vi "Drive Controller.vi"(8 "error in":errorcluster) -> ()   [LabVIEW 2020]
doc: "This VI executes continuously carrying out the current operation and responding to updates or new operation requests. It will often contain the timing or control code that is difficult to place directly in TeleOp. This VI generally opens all sensors and motors and isolates the rest of the robot code from knowing implementation details of how the operations are carried out."
uses:
  Drive Operations.ctl
  Drive Setpoints.ctl
  <vilib>/Rock Robotics/WPI/SafetyOutput/WPI_SafetyOutputConfigMenu.ctl
  <vilib>/Rock Robotics/WPI/RobotDrive/WPI_RobotDriveOpen2MotorWithExistingMotors.vi
  <vilib>/Rock Robotics/WPI/Framework/Completion Status.ctl
panel:
  in  "Interactive Values":T1
  in  "Buttons":cluster{"Execute Cmd":bool, "Abort Cmd":bool}
  out "Command Timing":cluster{"Start Time (ms)":u32, "Iterations":i32}
  out "Status":T3
  out "Setpoints":T4(graph)
  out "Current\nCmd":string
  # "Tip: The graph shows the motor setpoints. It may also be helpful to observe inputs and sensor values.\nYou may also want to display tuning or debugging controls."
  # "Interactive Command: You may fill in the settings for a command\nand schedule it with the Execute button. You can observe and abort\nany command while fine tuning the code for the controller."
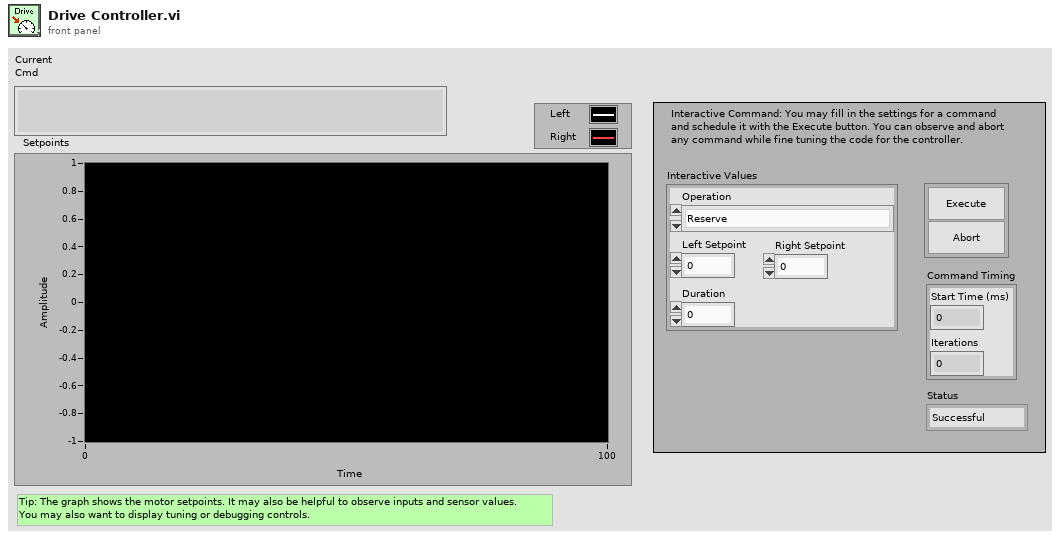
[diagram p1: front panel]
types:
  T1 = typedef "Drive Setpoints.ctl" = cluster{"Operation":T2, "Left Setpoint":dbl, "Right Setpoint":dbl, "Duration":dbl}
  T2 = typedef "Drive Operations.ctl" = enum16{"Reserve", "Read Current", "Immediate", "Drive for Time", "Drive for Distance"}
  T3 = typedef "Completion Status.ctl" = enum16{"Successful", "Aborted", "Incomplete"}
  T4 = cluster{"Left Setpoint":dbl, "Right Setpoint":dbl}
  T5 = typedef "WPI_SafetyOutputConfigMenu.ctl" = enum16{"Enable", "Disable"}
  T6 = typedef "WPI_MotorControlDeviceRef.ctl" = cluster{"DeviceStatus":errorcluster, "Type":T7, "PWM":cluster{"PWM Channel":T8, "DeadBand":T9}, "CAN":cluster{"Device Number":u8, "SetOutput VI Ref":variant, "GetOutput VI Ref":variant, "Enable VI Ref":variant, "Disable VI Ref":variant, "Data":variant}, "Invert":bool, "DIO PWM":cluster{"PWM \"Enable\" Channel":T8, "DIOChannel":T10, "PWM Rate":dbl}}
  T7 = typedef "WPI_MotorControlType.ctl" = enum16{"PWM", "CAN", "DIO PWM"}
  T8 = typedef "FPGA_DIOPWMChannel.ctl" = enum8{"PWM 0", "PWM 1", "PWM 2", "PWM 3", "PWM 4", "PWM 5", "PWM 6", "PWM 7", "PWM 8", "PWM 9", "PWM MXP 0", "PWM MXP 1", "PWM MXP 2", "PWM MXP 3", "PWM MXP 4", "PWM MXP 5", "PWM MXP 6", "PWM MXP 7", "PWM MXP 8", "PWM MXP 9", "Invalid"}
  T9 = typedef "WPI_PWMDeadband.ctl" = cluster{"Name":string, "maxPositivePwm":i32, "minPositivePwm":i32, "centerPwm":i32, "maxNegativePwm":i32, "minNegativePwm":i32, "angularRange":u16}
  T10 = typedef "FPGA_DIOChannel.ctl" = enum8{"DIO 0", "DIO 1", "DIO 2", "DIO 3", "DIO 4", "DIO 5", "DIO 6", "DIO 7", "DIO 8", "DIO 9", "DIO MXP 0", "DIO MXP 1", "DIO MXP 2", "DIO MXP 3", "DIO MXP 4", "DIO MXP 5", "DIO MXP 6", "DIO MXP 7", "DIO MXP 8", "DIO MXP 9", "DIO MXP 10", "DIO MXP 11", "DIO MXP 12", "DIO MXP 13", "DIO MXP 14", "DIO MXP 15", "SPI Port CS1", "SPI Port CS2", "SPI Port CS3", "SPI Port MISO", "SPI Port MOSI", "Invalid"}
  T11 = typedef "WPI_RobotDriveDevRef.ctl" = cluster{"DevStatus":errorcluster, "Motors[]":T6[], "Square Inputs":bool, "Max Output":dbl}
  T12 = typedef "Command Status Info.ctl" = cluster{"Name":string, "Status":T3, "notifier out":T13}
  T13 = typedef "Completion Notifier.ctl" = refnum<notifier>
  T14 = cluster{"SubSystem Data":T1, cluster{"Start Time (ms)":u32, "Iterations":i32}, cluster{"Command Info":T12, "Description":string, "Default Command":T1, "queue out":refnum<queue>, "Subsystem Name":string}}
  T15 = cluster{"SubSystem Data":T1, cluster{"Start Time (ms)":u32, "Iterations":i32}, "Default Command Arguments":cluster{"Command Info":T12, "Description":string, "Default Command":T1, "queue out":refnum<queue>, "Subsystem Name":string}}
  T16 = cluster{"Don't move motors while reserved":dbl, "Don't move motors while reserved":dbl}
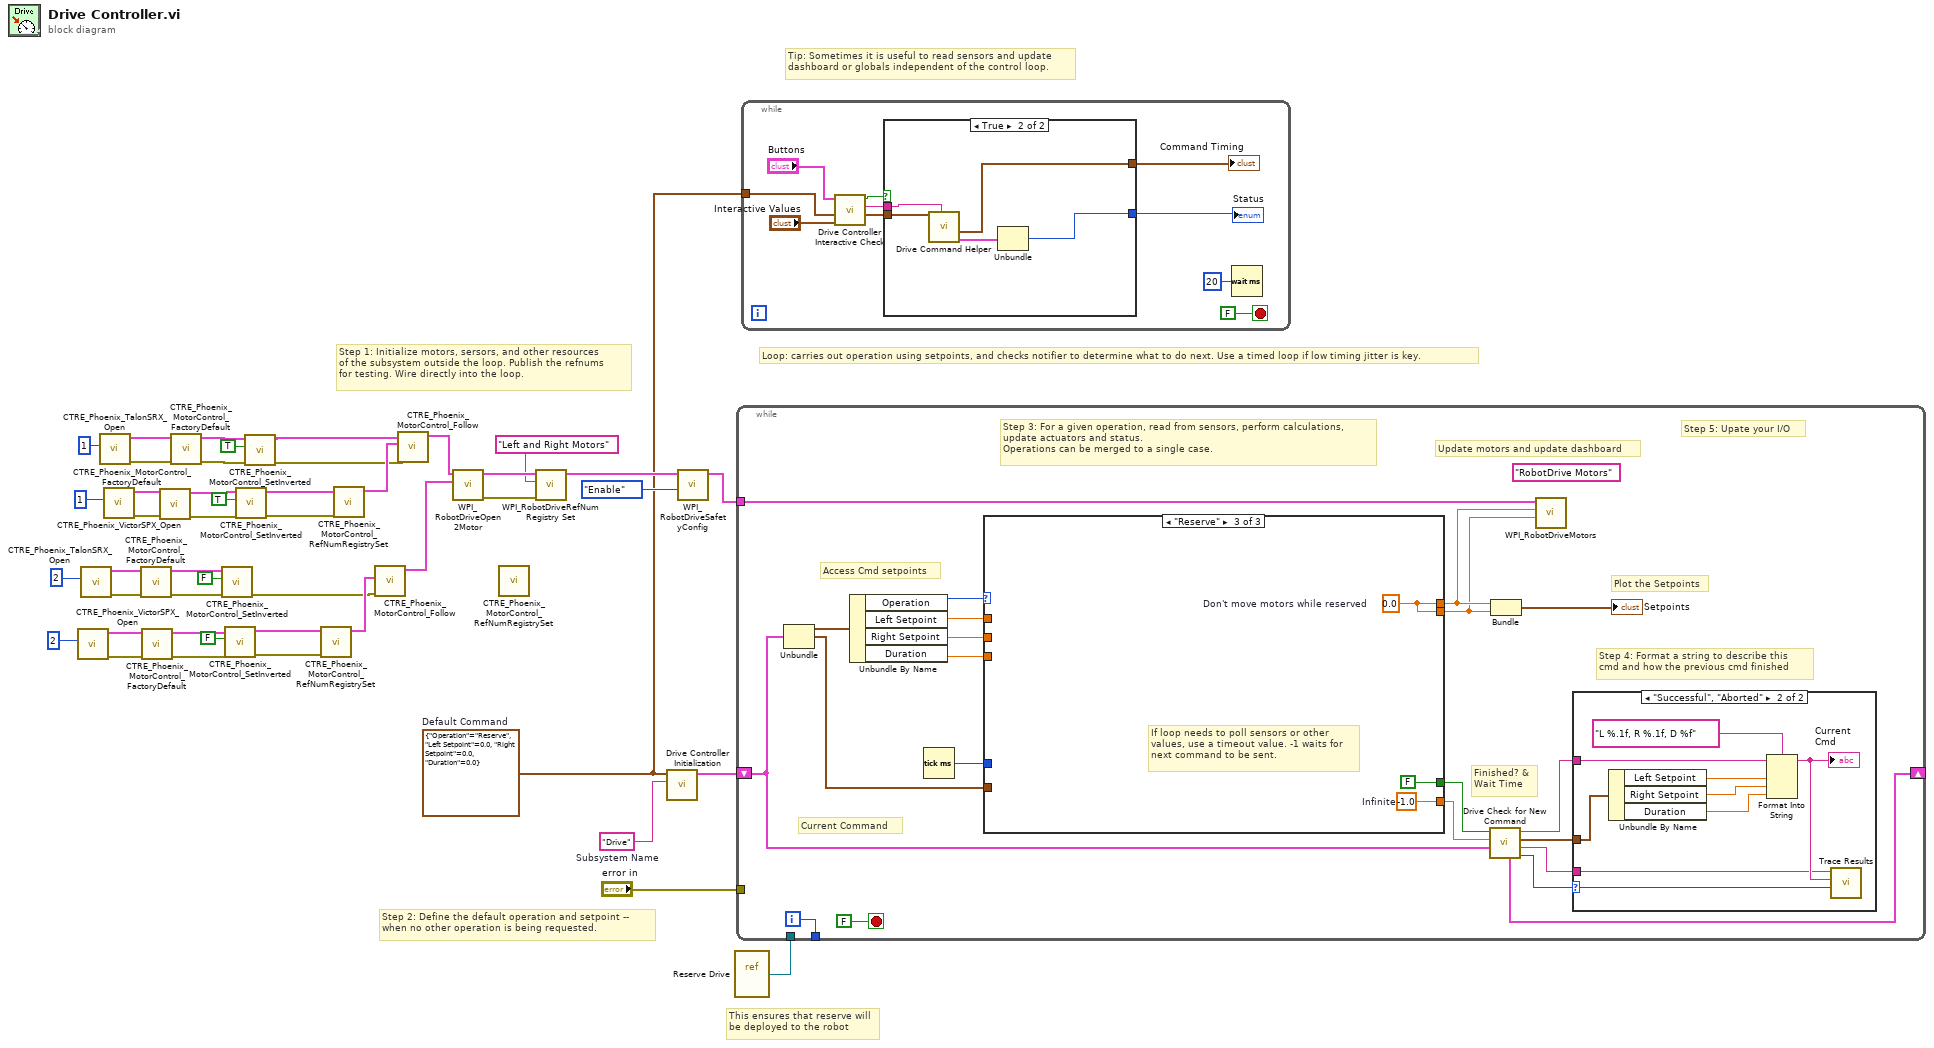
[diagram p0: block diagram]
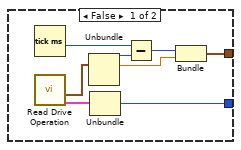
[diagram p2: hidden frame]
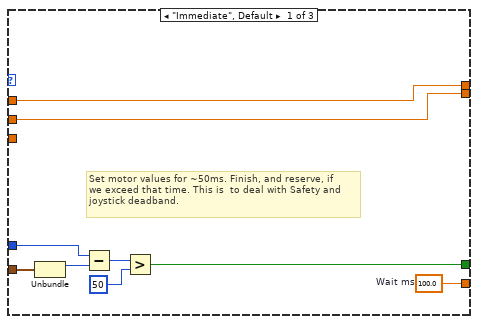
[diagram p4: hidden frame]
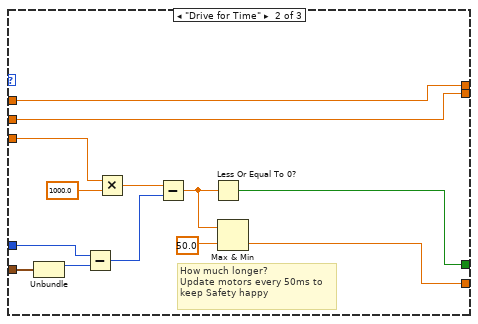
[diagram p5: hidden frame]
diagram:
  w36 = T1 {"Operation"=enum."Reserve", "Left Setpoint"=0.0, "Right Setpoint"=0.0, "Duration"=0.0}  # Default Command
  w46 = "Drive"  # Subsystem Name
  # "This ensures that reserve will\nbe deployed to the robot"
  # "Tip: Sometimes it is useful to read sensors and update\ndashboard or globals independent of the control loop."
  # "Step 2: Define the default operation and setpoint --\nwhen no other operation is being requested."
  # "Step 1: Initialize motors, sersors, and other resources\nof the subsystem outside the loop. Publish the refnums\nfor testing. Wire directly into the loop."
  # "Loop: carries out operation using setpoints, and checks notifier to determine what to do next. Use a timed loop if low timing jitter is key."
  n1 = call <vilib>:"CTRE_Phoenix_VictorSPX_Open.vi"("Device Number"=u8 2) -> ("error out"=w29:errorcluster, "PhoenixMotorControlDevRef"=w28:T6)  [unwired: 9 in]
  n2 = call <vilib>:"CTRE_Phoenix_TalonSRX_Open.vi"("Device Number"=u8 2) -> ("error out"=w24:errorcluster, "PhoenixMotorControlDevRef"=w30:T6)  [unwired: 9 in]
  n3 = call <vilib>:"CTRE_Phoenix_TalonSRX_Open.vi"("Device Number"=u8 1) -> ("error out"=w23:errorcluster, "PhoenixMotorControlDevRef"=w31:T6)  [unwired: 9 in]
  n4 = call <vilib>:"CTRE_Phoenix_VictorSPX_Open.vi"("Device Number"=u8 1) -> ("error out"=w25:errorcluster, "PhoenixMotorControlDevRef"=w26:T6)  [unwired: 9 in]
  n5 = call <vilib>:"CTRE_Phoenix_MotorControl_FactoryDefault.vi"("error in"=w24, "PhoenixMotorControlDevRef"=w30) -> ("error out"=w14:errorcluster, "PhoenixMotorControlDevRef"=w15:T6)  [unwired: 8 in]
  n6 = call <vilib>:"CTRE_Phoenix_MotorControl_FactoryDefault.vi"("error in"=w29, "PhoenixMotorControlDevRef"=w28) -> ("error out"=w12:errorcluster, "PhoenixMotorControlDevRef"=w13:T6)  [unwired: 8 in]
  n7 = call <vilib>:"CTRE_Phoenix_MotorControl_FactoryDefault.vi"("error in"=w25, "PhoenixMotorControlDevRef"=w26) -> ("error out"=w19:errorcluster, "PhoenixMotorControlDevRef"=w20:T6)  [unwired: 8 in]
  n8 = call <vilib>:"CTRE_Phoenix_MotorControl_FactoryDefault.vi"("error in"=w23, "PhoenixMotorControlDevRef"=w31) -> ("error out"=w21:errorcluster, "PhoenixMotorControlDevRef"=w22:T6)  [unwired: 8 in]
  n9 = call <vilib>:"CTRE_Phoenix_MotorControl_SetInverted.vi"("error in (no error)"=w14, "Invert?"=FALSE, "PhoenixMotorControlDevRef"=w15) -> ("error out"=w2:errorcluster)  [unwired: 7 in, 1 out]
  n10 = call <vilib>:"CTRE_Phoenix_MotorControl_SetInverted.vi"("error in (no error)"=w12, "Invert?"=FALSE, "PhoenixMotorControlDevRef"=w13) -> ("error out"=w8:errorcluster, "PhoenixMotorControlDevRef"=w9:T6)  [unwired: 7 in]
  n11 = call <vilib>:"CTRE_Phoenix_MotorControl_SetInverted.vi"("error in (no error)"=w19, "Invert?"=TRUE, "PhoenixMotorControlDevRef"=w20) -> ("error out"=w17:errorcluster, "PhoenixMotorControlDevRef"=w1:T6)  [unwired: 7 in]
  n12 = call <vilib>:"CTRE_Phoenix_MotorControl_SetInverted.vi"("error in (no error)"=w21, "Invert?"=TRUE, "PhoenixMotorControlDevRef"=w22) -> ("error out"=w3:errorcluster, "PhoenixMotorControlDevRef"=w7:T6)  [unwired: 7 in]
  n13 = call <vilib>:"CTRE_Phoenix_MotorControl_RefNumRegistrySet.vi"("error in (no error)"=w8, "PhoenixMotorControlDevRef"=w9) -> ("PhoenixMotorControlDevRef"=w27:T6)  [unwired: 8 in, 1 out]
  n14 = call <vilib>:"CTRE_Phoenix_MotorControl_RefNumRegistrySet.vi"("error in (no error)"=w17, "PhoenixMotorControlDevRef"=w1) -> ("PhoenixMotorControlDevRef"=w4:T6)  [unwired: 8 in, 1 out]
  n15 = call <vilib>:"CTRE_Phoenix_MotorControl_Follow.vi"("error in (no error)"=w2, "Master Controller to Follow"=w27) -> ("PhoenixMotorControlDevRef"=w5:T6)  [unwired: 8 in, 1 out]
  n16 = call <vilib>:"CTRE_Phoenix_MotorControl_Follow.vi"("error in (no error)"=w3, "Master Controller to Follow"=w4, "PhoenixMotorControlDevRef"=w7) -> ("PhoenixMotorControlDevRef"=w6:T6)  [unwired: 7 in, 1 out]
  n17 = call-poly <vilib>:"WPI_RobotDriveOpen2Motor.vi"("Right Motor Dev Ref"=w5, "Left Motor Dev Ref"=w6) -> ("error out"=w43:errorcluster, "RobotDriveDevRef"=w45:T11)  [unwired: 3 in, 5 out]
  n18 = call <vilib>:"CTRE_Phoenix_MotorControl_RefNumRegistrySet.vi"() -> ()  [unwired: 10 in, 2 out]
  n19 = call <vilib>:"WPI_RobotDriveRefNum Registry Set.vi"("error in (no error)"=w43, "refnum name"="Left and Right Motors", "RobotDriveDevRef"=w45) -> ("RobotDriveDevRef"=w42:T11)  [unwired: 1 in, 7 out]
  n20 = call "Drive Controller Initialization.vi"("Subsystem Name"=w46, "Default Command"=w36) -> ("Current Command"=w38:T14)  [unwired: 9 in]
  n21 = call <vilib>:"WPI_RobotDriveSafetyConfig.vi"("mode"=WPI_SafetyOutputConfigMenu."Enable", "RobotDriveDevRef"=w42) -> ("RobotDriveDevRef"=w40:T11)  [unwired: 8 in, 1 out]
  n22 = vi-ref "Reserve Drive.vi"() -> (w37:refnum<vi>)
  n23 = while {
    shift-right: [w54] -> _
    shift-left: w38 -> [w47]
    tunnel: [w66] -> _
    tunnel: w40 -> [w62]
    tunnel: "error in" -> [_]
    tunnel: w37 -> [_]
    i -> [w66]
    stop <- FALSE stop-if-true
    (unwired) "RobotDrive Motors" ("Name")
    # "Step 5: Upate your I/O"
    # "Step 4: Format a string to describe this\ncmd and how the previous cmd finished"
    # "Current Command"
    # "Update motors and update dashboard"
    # "Plot the Setpoints"
    # "Access Cmd setpoints"
    # "Finished? &\nWait Time"
    # "Step 3: For a given operation, read from sensors, perform calculations,\nupdate actuators and status.\nOperations can be merged to a single case."
    n24 = Unbundle(w47) -> ("SubSystem Data"=w61:T1, w48:cluster{"Start Time (ms)":u32, "Iterations":i32})  [unwired: 1 out]
    n25 = Unbundle By Name(w61) -> ("Operation"=w60:T2, "Left Setpoint"=w59:dbl, "Right Setpoint"=w58:dbl, "Duration"=w57:dbl)
    n26 = Tick Count (ms)() -> (millisecond timer value=w56:u32)
    n27 = case shown="\"Reserve\"" w60 {
      tunnel: [w85 w86 w101] -> w53
      tunnel: [w78 w93 FALSE ("ignore previous (F)")] -> w52
      tunnel: w48 -> [w77 w95 _]
      tunnel: [w84 w92 w99] -> w64
      tunnel: [w83 w91 w99] -> w63
      tunnel: w59 -> [w84 w92 _]
      tunnel: w58 -> [w83 w91 _]
      tunnel: w57 -> [_ w90 _]
      tunnel: w56 -> [w79 w89 _]
      frame "Immediate", Default {
        w85 = 100.0  # Wait ms
        # "Set motor values for ~50ms. Finish, and reserve, if\nwe exceed that time. This is  to deal with Safety and\njoystick deadband."
        n28 = Unbundle(w77) -> ("Start Time (ms)"=w80:u32)  [unwired: 1 out]
        n29 = Subtract(x=w79, y=w80) -> (x-y=w81:u32)
        n30 = Greater?(x=w81, y=u8 50 ("Left Motor")) -> (0:w78:bool)
      }
      frame "Drive for Time" {
        # "How much longer?\nUpdate motors every 50ms to\nkeep Safety happy"
        n31 = Unbundle(w95) -> ("Start Time (ms)"=w94:u32)  [unwired: 1 out]
        n32 = Subtract(x=w89, y=w94) -> (x-y=w98:u32)
        n33 = Multiply(x=w90, y=1000.0) -> (x*y=w97:dbl)
        n34 = Subtract(x=w97, y=w98) -> (x-y=w88:dbl)
        n35 = Less Or Equal To 0?(x=w88) -> (x <= 0?=w93:bool)
        n36 = Max & Min(x=w88, y=50.0) -> (min(x,y)=w86:dbl)  [unwired: 1 out]
      }
      frame "Reserve" {
        w99 = 0.0  # Don't move motors while reserved
        w101 = -1.0  # Infinite
        # "If loop needs to poll sensors or other\nvalues, use a timeout value. -1 waits for\nnext command to be sent."
      }
    }
    n37 = call "Drive Check for New Command.vi"("input cluster"=w47, "Wait time (ms)"=w53, "Finished?"=w52) -> ("Completion"=w55:T3, "Subsystem Name"=w49:string, "Current Command"=w50:T1, "Initial Trace String"=w51:string, "Next Command"=w54:T15)  [unwired: 4 in]
    n38 = Bundle("Don't move motors while reserved"=w64, "Don't move motors while reserved"=w63) -> (→"Setpoints":T16)  [unwired: 1 in]
    n39 = call <vilib>:"WPI_RobotDriveMotors.vi"("RightSpeed"=w63, "LeftSpeed"=w64, "RobotDriveDevRef"=w62) -> ()  [unwired: 1 in, 8 out]
    n40 = case shown="\"Successful\", \"Aborted\"" w55 {
      selector: w55 -> [_ w76]
      tunnel: w51 -> [_ w71]
      tunnel: w50 -> [_ w72]
      tunnel: w49 -> [_ w68]
      frame "Incomplete", Default {
        # "Continuing current command"
      }
      frame "Successful", "Aborted" {
        # "Report and setup for next command"
        n41 = Unbundle By Name(w72) -> ("Left Setpoint"=w74:dbl, "Right Setpoint"=w75:dbl, "Duration"=w69:dbl)
        n42 = Format Into String(format string="L %.1f, R %.1f, D %f", initial string=w71, w74, w75, w69) -> (resulting string=w70:string)  [unwired: 1 in, 1 out]
        "Current\nCmd" <- w70
        n43 = call <vilib>:"Trace Results.vi"("Status of previous command"=w76, "Description"=w70, "Subsystem"=w68) -> ()  [unwired: 9 in]
      }
    }
  }
  n44 = while {
    tunnel: w36 -> [w103]
    stop <- FALSE stop-if-true
    n45 = call "Drive Controller Interactive Check.vi"("Interactive Command In"="Interactive Values", "Default Command"=w103, "Buttons"="Buttons") -> ("Interactive Command Out"=w105:T1, "Trace String"=w106:string, "Schedule"=w107:bool)  [unwired: 6 in]
    n46 = case shown="True" w107 {
      tunnel: [w116 w124] -> w108
      tunnel: [w115 w120] -> w109
      tunnel: w106 -> [_ w122]
      tunnel: w105 -> [_ w121]
      frame False {
        n47 = Tick Count (ms)() -> (millisecond timer value=w119:u32)
        n48 = call "Read Drive Operation.vi"() -> ("Command Info"=w113:T12, "SubSystem Data"=w112:T1)  [unwired: 9 in, 1 out]
        n49 = Unbundle(w112) -> ("Operation"=w117:T2, "Left Setpoint"=w114:dbl)  [unwired: 2 out]
        n50 = Unbundle(w113) -> ("Status"=w116:T3)  [unwired: 2 out]
        n51 = Subtract(x=w119, y=w117) -> (x-y=w118:u32)
        n52 = Bundle(w118, "Left Setpoint"=w114) -> (w115:cluster{u32, "Left Setpoint":dbl})  [unwired: 1 in]
      }
      frame True {
        n53 = call "Drive Command Helper.vi"("Description"=w122, "SubSystem Data"=w121) -> ("Command Info Out"=w123:T12, "Command Timing"=w120:cluster{"Start Time (ms)":u32, "Iterations":i32})  [unwired: 7 in, 1 out]
        n54 = Unbundle(w123) -> ("Status"=w124:T3)  [unwired: 2 out]
      }
    }
    "Status" <- w108
    "Command Timing" <- w109
    n55 = Wait (ms)(milliseconds to wait=u32 20) -> ()  [unwired: 1 out]
  }
